vi "[WLC] Calculate Force.vi"(1 "Temperature (K)":dbl=298.0, 2 "Persistence Length (nm)":dbl, 3 "Contour Length (nm)":dbl, 4 "Extension (nm)":dbl) -> (0 "Force (pN)":dbl)   [LabVIEW 2013]
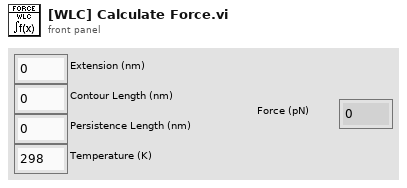
[diagram p1: front panel]
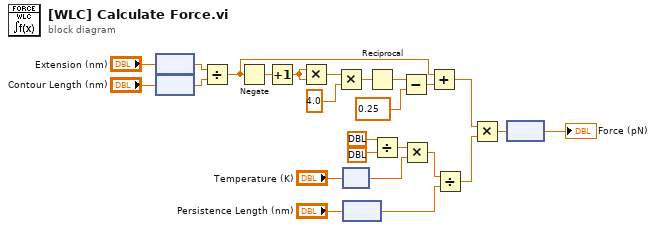
[diagram p0: block diagram]
diagram:
  n1 = node("Extension (nm)") -> (w14:dbl[unit])
  n2 = node("Contour Length (nm)") -> (w15:dbl[unit])
  n3 = Divide(x=w14, y=w15) -> (x/y=w5:dbl)
  n4 = Negate(x=w5) -> (-x=w13:dbl)
  n5 = Increment(x=w13) -> (x+1=w12:dbl)
  n6 = Multiply(x=w12, y=w12) -> (x*y=w11:dbl)
  n7 = Multiply(x=w11, y=4.0) -> (x*y=w9:dbl)
  n8 = node("Temperature (K)") -> (w25:dbl[unit])
  n9 = node("Persistence Length (nm)") -> (w18:dbl[unit])
  n10 = Reciprocal(x=w9) -> (1/x=w8:dbl)
  n11 = Divide(x=ext[unit] 8.314472, y=ext[unit] 6.0221415e+23) -> (x/y=w23:ext[unit])
  n12 = Subtract(x=w8, y=0.25) -> (x-y=w6:dbl)
  n13 = Multiply(x=w23, y=w25) -> (x*y=w19:ext[unit])
  n14 = Add(x=w5, y=w6) -> (x+y=w2:dbl)
  n15 = Divide(x=w19, y=w18) -> (x/y=w1:ext[unit])
  n16 = Multiply(x=w2, y=w1) -> (x*y=w4:ext[unit])
  n17 = node(w4) -> (→"Force (pN)":ext)
